vi "Get Minimum LabVIEW Version.vi"(8 "error in (no error)":errorcluster, 11 "9224 in":refnum<class "9224.lvclass">) -> (0 "error out":errorcluster, 2 "Minimum LabVIEW Version":i32, 3 "9224 out":refnum<class "9224.lvclass">)   [LabVIEW 2019, in "Modules.lvlib" / "9224.lvclass"]
uses:
  9224.lvclass
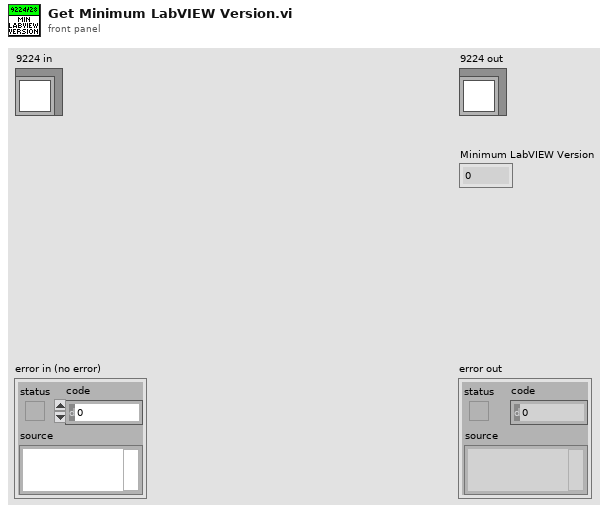
[diagram p1: front panel]
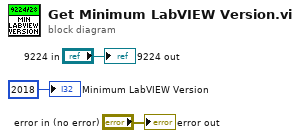
[diagram p0: block diagram]
diagram:
  "error out" <- "error in (no error)"
  "9224 out" <- "9224 in"
  "Minimum LabVIEW Version" <- 2018 ("Minimum LabVIEW Version")
